vi "Send_UIStop.vi"(6 "HighPriority (F)":bool, 8 "error in":errorcluster, 11 "Queue in":refnum<queue>) -> (0 "error out":errorcluster)   [LabVIEW 2018, in "UI_Library.lvlib"]
uses:
  UI_Library.lvlib
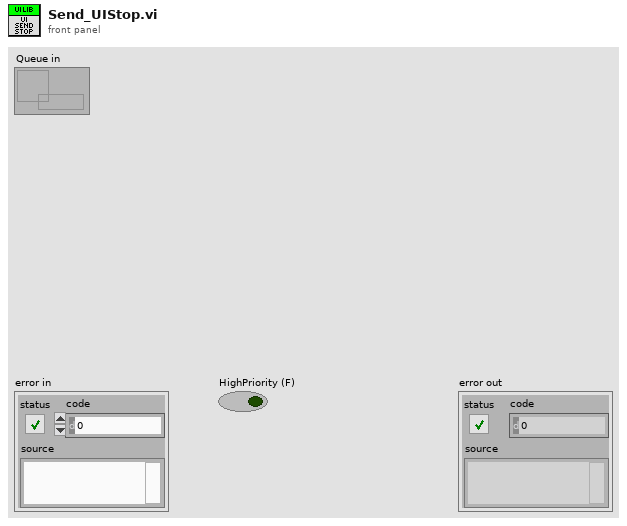
[diagram p1: front panel]
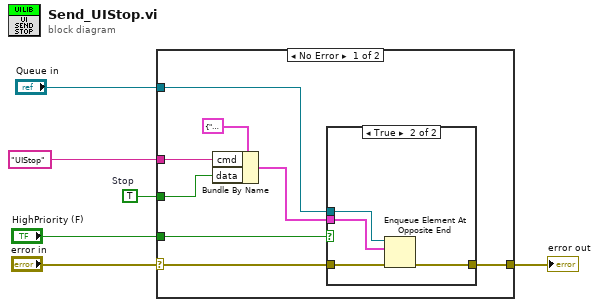
[diagram p0: block diagram]
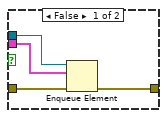
[diagram p2: hidden frame]
diagram:
  w2 = TRUE  # Stop
  n1 = case shown="No Error" "error in" {
    selector: "error in" -> [w8 w23]
    tunnel: "Queue in" -> [w14 _]
    tunnel: w2 -> [w11 _]
    tunnel: "UIStop" ("UICmd") -> [w10 _]
    tunnel: "HighPriority (F)" -> [w9 _]
    tunnel: [w7 w23] -> w6
    frame No Error {
      n2 = Bundle By Name(cluster=cluster{"cmd":string, "data":variant} {"cmd"="", "data"=variant} ("element"), "cmd"=w10, "data"=w11) -> (w12:cluster{"cmd":string, "data":variant})
      n3 = case shown="True" w9 {
        tunnel: w14 -> [w18 w21]
        tunnel: w12 -> [w17 w20]
        tunnel: w8 -> [w16 w22]
        tunnel: [w15 w19] -> w7
        frame False {
          n4 = Enqueue Element(queue=w18, element=w17, error in (no error)=w16) -> (error out=w15:errorcluster)  [unwired: 1 in, 2 out]
        }
        frame True {
          n5 = Enqueue Element At Opposite End(queue=w21, element=w20, error in (no error)=w22) -> (error out=w19:errorcluster)  [unwired: 1 in, 2 out]
        }
      }
    }
    frame Error {
    }
  }
  "error out" <- w6
